vi "MALT132 set several output.vi"() -> ()   [LabVIEW 2018]
uses:
  <instrlib>/AltonTech MALT/AltonTech MALT200817.lvlib
panel:
  in  "Clr 0xAA":bool
  in  "Clr 0x55":bool
  in  "Address":i32=4 format="%02x"
  in  "Set 0x55":bool
  in  "Set 0xAA":bool
  in  "stop":bool
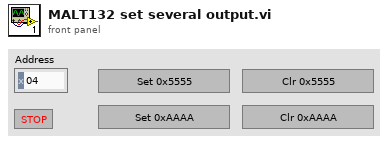
[diagram p1: front panel]
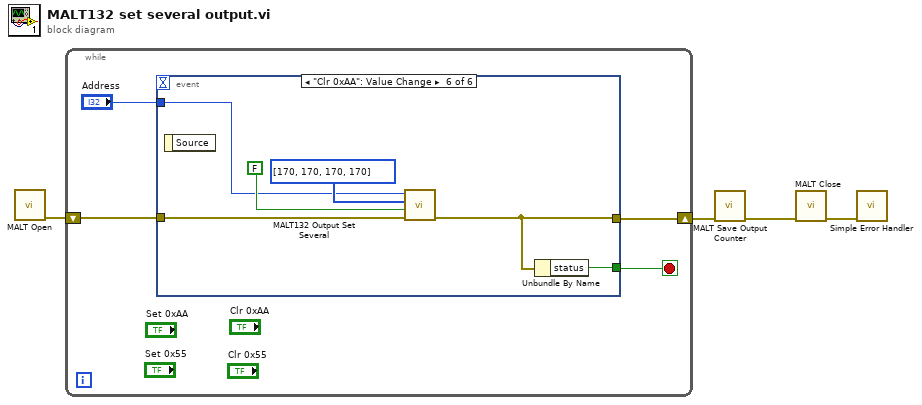
[diagram p0: block diagram]
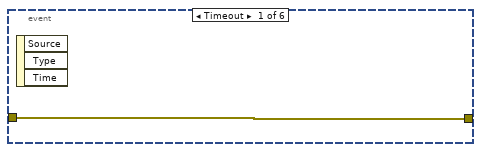
[diagram p2: hidden frame]
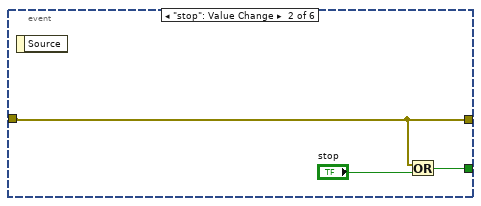
[diagram p3: hidden frame]
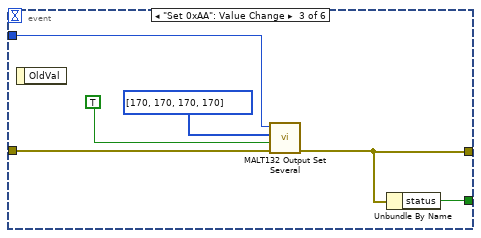
[diagram p4: hidden frame]
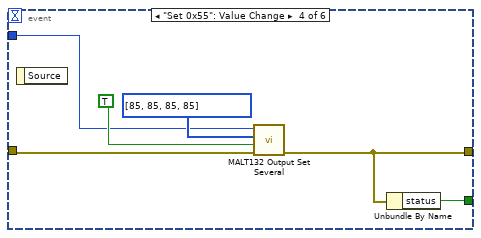
[diagram p5: hidden frame]
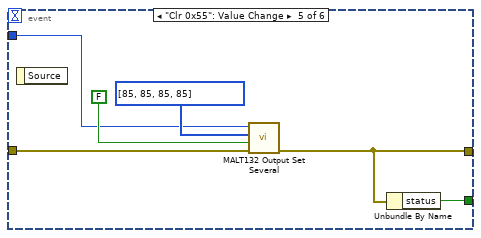
[diagram p6: hidden frame]
diagram:
  n1 = call <instrlib>:"MALT Open.vi"() -> ("error out"=w4:errorcluster)  [unwired: 10 in, 1 out]
  n2 = while {
    shift-right: [w7] -> w2
    shift-left: w4 -> [w8]
    stop <- w6 stop-if-true
    n3 = event shown="[5] \"Clr 0xAA\": Value Change" {
      selector: _ -> [_ _ _ _ _ _]
      dyn-events: _ -> [_ _ _ _ _ _]
      timeout: _ -> [_ _ _ _ _ _]
      tunnel: w8 -> [w9 w10 w16 w22 w28 w34]
      tunnel: [w9 w10 w14 w20 w26 w32] -> w7
      tunnel: [_ w12 w15 w21 w27 w33] -> w6
      tunnel: "Address" -> [_ _ w13 w19 w25 w31]
      event Timeout {
        n4 = event-data() -> ()  [unwired: 1 in, 3 out]
      }
      event "stop": Value Change {
        n5 = event-data() -> ()  [unwired: 1 in, 1 out]
        n6 = Or(x=w10, y="stop") -> (x .or. y?=w12:bool)
      }
      event "Set 0xAA": Value Change {
        n7 = event-data() -> ()  [unwired: 1 in, 1 out]
        n8 = call <instrlib>:"MALT132 Output Set Several.vi"("error in"=w16, "State"=TRUE, "State Map"=u8[] [170, 170, 170, 170], "Address"=w13) -> ("error out"=w14:errorcluster)  [unwired: 7 in]
        n9 = Unbundle By Name(w14) -> ("status"=w15:bool)
      }
      event "Set 0x55": Value Change {
        n10 = event-data() -> ()  [unwired: 1 in, 1 out]
        n11 = call <instrlib>:"MALT132 Output Set Several.vi"("error in"=w22, "State"=TRUE, "State Map"=u8[] [85, 85, 85, 85], "Address"=w19) -> ("error out"=w20:errorcluster)  [unwired: 7 in]
        n12 = Unbundle By Name(w20) -> ("status"=w21:bool)
      }
      event "Clr 0x55": Value Change {
        n13 = event-data() -> ()  [unwired: 1 in, 1 out]
        n14 = call <instrlib>:"MALT132 Output Set Several.vi"("error in"=w28, "State"=FALSE, "State Map"=u8[] [85, 85, 85, 85], "Address"=w25) -> ("error out"=w26:errorcluster)  [unwired: 7 in]
        n15 = Unbundle By Name(w26) -> ("status"=w27:bool)
      }
      event "Clr 0xAA": Value Change {
        n16 = event-data() -> ()  [unwired: 1 in, 1 out]
        n17 = call <instrlib>:"MALT132 Output Set Several.vi"("error in"=w34, "State"=FALSE, "State Map"=u8[] [170, 170, 170, 170], "Address"=w31) -> ("error out"=w32:errorcluster)  [unwired: 7 in]
        n18 = Unbundle By Name(w32) -> ("status"=w33:bool)
      }
    }
  }
  n19 = call <instrlib>:"MALT Save Output Counter.vi"("error in"=w2) -> ("error out"=w1:errorcluster)  [unwired: 10 in]
  n20 = call <instrlib>:"MALT Close.vi"("error in"=w1) -> ("error out"=w3:errorcluster)  [unwired: 10 in]
  n21 = call <vilib>:"Simple Error Handler.vi"("error in (no error)"=w3) -> ()  [unwired: 4 in, 5 out]
